vi "SP Add Marker to Table.vi"(7 "CH Control In":T3={"Trace Orientation"=enum."Overlay", "Frequency"={"Change Frequency"=FALSE, "Start"=500.0, "Stop"=1500.0, "Units"=enum."MHz"}, "Markers"=[], "Traces"=[]} {"Traces"."Reference" format="%#.2g"; "Traces"."Display Data" items=["Data", "Memory", "Data/Memory"]; "Traces"."Format" items=["Log Mag", "Phase", "Expanded Phase", "Delay", "Smith", "Polar", "Lin Mag", "SWR", "Loss", "Real", "Imaginary"]; "Traces"."Scale" min=0.001 step=1.0 format="%#.2g"; "Traces"."Position" min=0.0 max=10.0; "Frequency"."Stop" format="%.3g"; "Frequency"."Start" format="%.3g"}, 8 "error in (no error)":errorcluster, 9 "Marker":T1, 10 "Marker Table":refnum<vi>, 11 "Plot Ref":refnum<vi>) -> (0 "error out":errorcluster, 1 "Marker Added":i32, 5 "CH Control Out":T3={"Trace Orientation"=enum."Overlay", "Frequency"={"Change Frequency"=FALSE, "Start"=500.0, "Stop"=1500.0, "Units"=enum."MHz"}, "Markers"=[], "Traces"=[]} {"Traces"."Reference" format="%#.2g"; "Traces"."Display Data" items=["Data", "Memory", "Data/Memory"]; "Traces"."Format" items=["Log Mag", "Phase", "Expanded Phase", "Delay", "Smith", "Polar", "Lin Mag", "SWR", "Loss", "Real", "Imaginary"]; "Traces"."Scale" min=0.001 step=1.0 format="%#.2g"; "Traces"."Position" min=0.0 max=10.0; "Frequency"."Stop" format="%.3g"; "Frequency"."Start" format="%.3g"})   [LabVIEW 2011]
uses:
  TypeDefs/SP Display Plot Controls Cluster.ctl
  TypeDefs/SP Frequency Units.ctl
  TypeDefs/SP Marker Cluster.ctl
  TypeDefs/SP Marker Type.ctl
  TypeDefs/SP Display Trace Controls.ctl
  TypeDefs/SP Display Format.ctl
  TypeDefs/SP Display Data.ctl
panel:
  # "Div"
  # "Div"
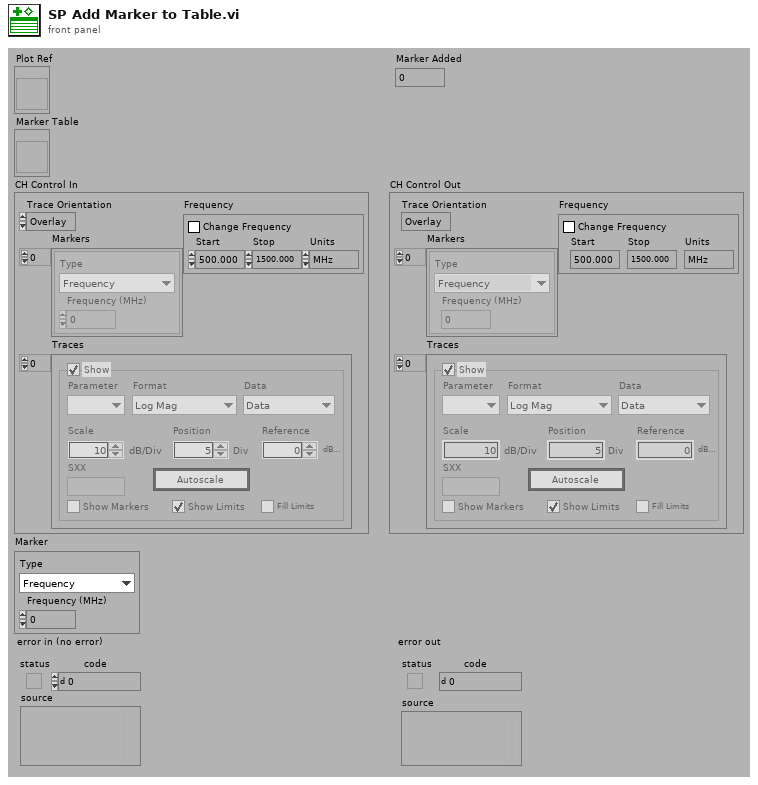
[diagram p1: front panel]
types:
  T1 = typedef "SP Marker Cluster.ctl" = cluster{"Type":T2, "Frequency (MHz)":dbl}
  T2 = typedef "SP Marker Type.ctl" = enum16{"Frequency", "Trace Maximum", "Trace Minimum", "Limit Maximum", "Limit Minimum"}
  T3 = typedef "SP Display Plot Controls Cluster.ctl" = cluster{"Trace Orientation":enum32{"Overlay", "Split"}, "Frequency":cluster{"Change Frequency":bool, "Start":dbl, "Stop":dbl, "Units":T4}, "Markers":T1[], "Traces":T5[]}
  T4 = typedef "SP Frequency Units.ctl" = enum16{"Hz", "kHz", "MHz", "GHz", "Points"}
  T5 = typedef "SP Display Trace Controls.ctl" = cluster{"Trace On":bool, "Measure":i32, "Format":T6, "Autoscale":bool, "Reference":dbl, "\nRefUnit":string, "Position":dbl, "Scale":dbl, "ScaleUnit":string, "LimitOn":bool, "LimitFill":bool, "Display Data":T7, "Show Markers":bool, "SXX":string}
  T6 = typedef "SP Display Format.ctl" = i32
  T7 = typedef "SP Display Data.ctl" = u16
  T8 = typedef "SP Channel Data.ctl" = cluster{"Graph Ref":refnum<vi>, "Data":cluster{"Data":cluster{"X":dbl[], "Y":dbl[]}, "Index":i32}, "ULimits":cluster{"Data":cluster{"X":dbl[], "Y":dbl[]}, "Index":i32}[], "LLimits":cluster{"Data":cluster{"X":dbl[], "Y":dbl[]}, "Index":i32}[]}
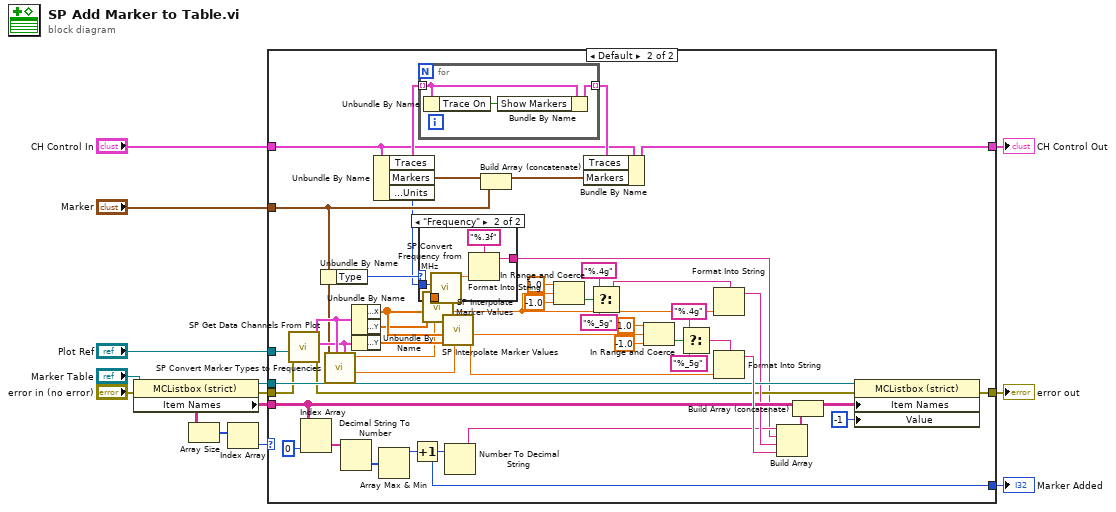
[diagram p0: block diagram]
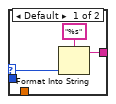
[diagram p3: hidden frame]
diagram:
  n1 = property class="MCListbox (strict)"(reference="Marker Table", error in="error in (no error)") -> (reference out=w9:refnum<vi>, error out=w10:errorcluster, "Item Names"=w7:string[][])
  n2 = Array Size(array=w7) -> (size(s)=w6:i32[])
  n3 = Index Array(array=w6) -> (element=w5:i32)  [unwired: 1 in]
  n4 = case shown="Default" w5 {
    tunnel: "Plot Ref" -> [_ w52]
    tunnel: w10 -> [w15 w51]
    tunnel: w9 -> [_ w58]
    tunnel: [w15 w57] -> w8
    tunnel: w7 -> [_ w55]
    tunnel: [_ w53] -> w4
    tunnel: "CH Control In" -> [w14 w42]
    tunnel: [w14 w49] -> w3
    tunnel: "Marker" -> [_ w34]
    frame 9.. {
      # "If there are already 8 markers, don't add anymore."
    }
    frame Default {
      n5 = call "SP Get Data Channels From Plot.vi"("error in (no error)"=w51, "Plot Ref"=w52) -> ("error out"=w50:errorcluster, "CH 2"=w36:T8, "CH 1"=w37:T8)  [unwired: 7 out]
      n6 = Index Array(array=w55, index (col)=0 ("disabled index (col)")) -> (element=w62:string[])  [unwired: 1 in]
      n7 = Unbundle By Name(w34) -> ("Type"=w33:T2)
      n8 = call "SP Convert Marker Types to Frequencies.vi"("CH 2"=w36, "CH 1"=w37, "Marker"=w34) -> ("CH2 Frequency"=w35:dbl, "CH1 Frequency"=w16:dbl)  [unwired: 5 out]
      n9 = Decimal String To Number(string=w62) -> (number=w61:i32[])  [unwired: 3 out]
      n10 = Unbundle By Name(w37) -> ("Data.Data.X"=w40:dbl[], "Data.Data.Y"=w39:dbl[])
      n11 = Unbundle By Name(w36) -> ("Data.Data.Y"=w41:dbl[])
      n12 = Unbundle By Name(w42) -> ("Traces"=w45:T5[], "Markers"=w38:T1[], "Frequency.Units"=w31:T4)
      n13 = Array Max & Min(array=w61) -> (max value=w47:i32)  [unwired: 3 out]
      n14 = Increment(x=w47) -> (x+1=w53:i32)
      n15 = for {
        tunnel: w45 -> [w74] mode=indexing
        tunnel: [w72] -> w44 mode=indexing
        n16 = Unbundle By Name(w74) -> ("Trace On"=w73:bool)
        n17 = Bundle By Name(cluster=w74, "Show Markers"=w73) -> (w72:T5)
      }
      n18 = case shown="\"Frequency\"" w33 {
        selector: w33 -> [w64 _]
        tunnel: [w65 w70] -> w32
        tunnel: w31 -> [_ w68]
        tunnel: w16 -> [_ w67]
        frame Default {
          n19 = Format Into String(format string="%s", w64) -> (resulting string=w65:string)  [unwired: 2 in, 1 out]
        }
        frame "Frequency" {
          n20 = call "SP Convert Frequency from MHz.vi"("Units"=w68, "Frequency (MHz)"=w67) -> ("Converted Frequency"=w69:dbl)  [unwired: 1 in, 8 out]
          n21 = Format Into String(format string="%.3f", w69) -> (resulting string=w70:string)  [unwired: 2 in, 1 out]
        }
      }
      n22 = call "SP Interpolate Marker Values.vi"("Marker Value"=w16, "Y Values"=w39, "X Values"=w40) -> ("Interpolated Y Value"=w18:dbl)  [unwired: 8 out]
      n23 = call "SP Interpolate Marker Values.vi"("Marker Value"=w35, "Y Values"=w41, "X Values"=w40) -> ("Interpolated Y Value"=w17:dbl)  [unwired: 8 out]
      n24 = Number To Decimal String(number=w53) -> (decimal integer string=w43:string)  [unwired: 1 out]
      n25 = Build Array (concatenate)(w38, w34) -> (w48:T1[])
      n26 = In Range and Coerce(upper limit=1.0, x=w18, lower limit=-1.0) -> (In Range?=w27:bool)  [unwired: 1 out]
      n27 = Bundle By Name(cluster=w42, "Traces"=w44, "Markers"=w48) -> (w49:T3)
      n28 = Select(t="%.4g" ("format string"), s=w27, f="%_5g" ("format string")) -> (s? t:f=w20:string)
      n29 = In Range and Coerce(upper limit=1.0, x=w17, lower limit=-1.0) -> (In Range?=w24:bool)  [unwired: 1 out]
      n30 = Select(t="%.4g" ("format string"), s=w24, f="%_5g" ("format string")) -> (s? t:f=w19:string)
      n31 = Format Into String(format string=w20, w18) -> (resulting string=w54:string)  [unwired: 2 in, 1 out]
      n32 = Format Into String(format string=w19, w17) -> (resulting string=w60:string)  [unwired: 2 in, 1 out]
      n33 = Build Array(w43, w32, w54, w60) -> (w59:string[])
      n34 = Build Array (concatenate)(w55, w59) -> (w56:string[][])
      n35 = property class="MCListbox (strict)"(reference=w58, error in=w50, "Item Names"=w56, "Value"=-1 ("Value (Signaling)")) -> (error out=w57:errorcluster)  [unwired: 1 out]
    }
  }
  "error out" <- w8
  "Marker Added" <- w4
  "CH Control Out" <- w3
